vi "Configure Stream U3.vi"(4 "Scan List (-)":u8[](array[numeric])=[31, 31, 31, 31, 31, 31, 31, 31, 31, 31, 31, 31, 31, 31, 31, 31, 31, 31, 31, 31, 31, 31, 31, 31, 31, 31, 31, 31, 31, 31, 31, 31, 31, 31, 31, 31, 31, 31, 31, 31, 31, 31, 31, 31, 31, 31, 31, 31, 31, 31, 31, 31, 31, 31, 31, 31, 31, 31, 31, 31, 31, 31, 31, 31, 31, 31, 31, 31, 31, 31, 31, 31, 31, 31, 31, 31, 31, 31, 31, 31, 31, 31, 31, 31, 31, 31, 31, 31, 31, 31, 31, 31, 31, 31, 31, 31, 31, 31, 31, 31, 31, 31, 31, 31, 31, 31, 31, 31, 31, 31, 31, 31, 31, 31, 31, 31, 31, 31, 31, 31, 31, 31, 31, 31, 31, 31, 31, 31], 6 "Wait Mode":string="LJ_swNONE", 7 "PC buffer size (seconds)":dbl=5.0 format="%.2f", 8 "error in":errorcluster, 9 "Scan List (+)":u8[](array[numeric])=[0, 1, 2, 3], 10 "Scan Rate (Hz)":dbl=1000.0 format="%.2f", 11 "Handle In":i32) -> (0 "error out":errorcluster, 2 "PC buffer size (samples)":i32=5, 3 "Handle Out":i32)   [LabVIEW 2021]
panel:
  # "The + scan list is the positive\nchannels.  For each element in\nthe + list, there must also be\nan element in the - list, which is\nthe negative channels.  For\nsingle-ended channels, put in\n31 for the negative channel."
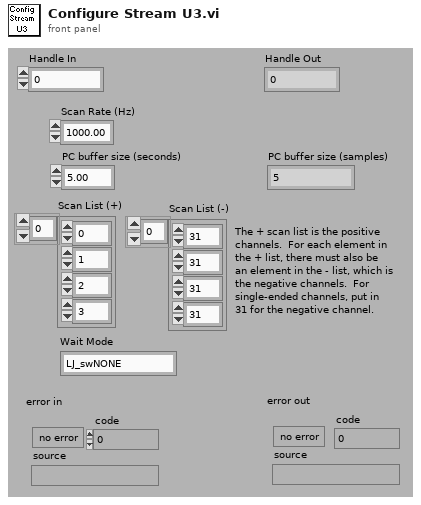
[diagram p1: front panel]
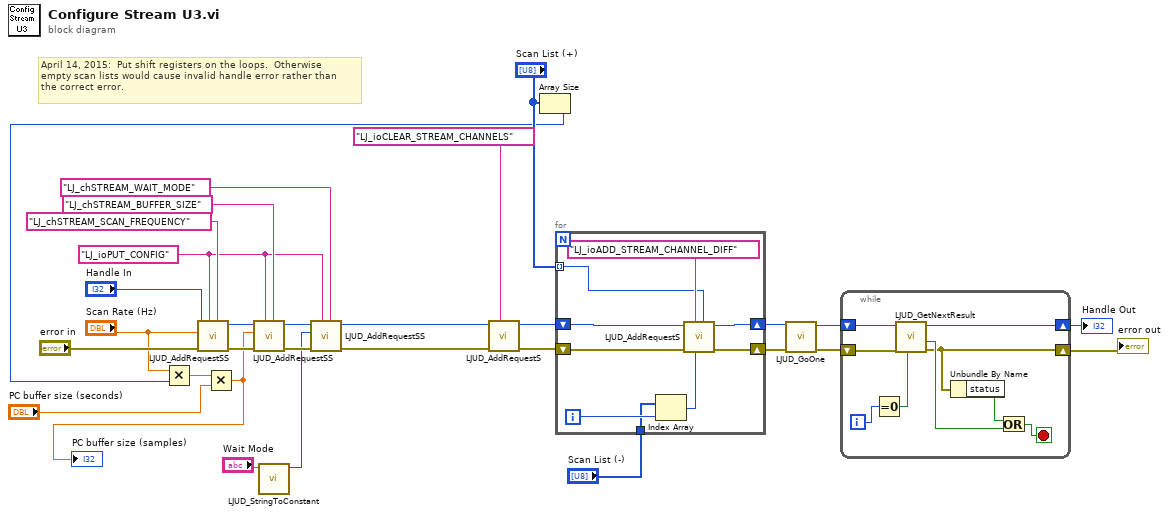
[diagram p0: block diagram]
diagram:
  w9 = "LJ_ioPUT_CONFIG" ("IOType")
  # "April 14, 2015:  Put shift registers on the loops.  Otherwise\nempty scan lists would cause invalid handle error rather than\nthe correct error."
  n1 = call "LJUD_AddRequestSS.vi"("Channel"="LJ_chSTREAM_SCAN_FREQUENCY" ("IOType"), "IOType"=w9, "error in"="error in", "Value"="Scan Rate (Hz)", "Handle In"="Handle In") -> ("error out"=w26:errorcluster, "Handle Out"=w28:i32)  [unwired: 5 in]
  n2 = call "LJUD_StringToConstant.vi"("String"="Wait Mode") -> ("Constant Number"=w7:i32)  [unwired: 9 in, 1 out]
  n3 = Array Size(array="Scan List (+)") -> (size(s)=w11:i32)
  n4 = Multiply(x="Scan Rate (Hz)", y=w11) -> (x*y=w16:dbl)
  n5 = Multiply(x=w16, y="PC buffer size (seconds)") -> (x*y=w4:dbl)
  "PC buffer size (samples)" <- w4
  n6 = call "LJUD_AddRequestSS.vi"("Channel"="LJ_chSTREAM_BUFFER_SIZE" ("IOType"), "IOType"=w9, "error in"=w26, "Value"=w4, "Handle In"=w28) -> ("error out"=w25:errorcluster, "Handle Out"=w27:i32)  [unwired: 5 in]
  n7 = call "LJUD_AddRequestSS.vi"("Channel"="LJ_chSTREAM_WAIT_MODE" ("IOType"), "IOType"=w9, "error in"=w25, "Value"=w7, "Handle In"=w27) -> ("error out"=w2:errorcluster, "Handle Out"=w3:i32)  [unwired: 5 in]
  n8 = call "LJUD_AddRequestS.vi"("IOType"="LJ_ioCLEAR_STREAM_CHANNELS", "error in"=w2, "Handle In"=w3) -> ("error out"=w14:errorcluster, "Handle Out"=w15:i32)  [unwired: 7 in]
  n9 = for {
    shift-right: [w36] -> w20
    shift-left: w14 -> [w37]
    tunnel: "Scan List (+)" -> [w34] mode=indexing
    tunnel: "Scan List (-)" -> [w32]
    shift-right: [w35] -> w21
    shift-left: w15 -> [w39]
    i -> [w33]
    n10 = Index Array(array=w32, index=w33) -> (element=w31:u8)
    n11 = call "LJUD_AddRequestS.vi"("Channel"=w34, "x1"=w31, "IOType"="LJ_ioADD_STREAM_CHANNEL_DIFF", "error in"=w37, "Handle In"=w39) -> ("error out"=w36:errorcluster, "Handle Out"=w35:i32)  [unwired: 5 in]
  }
  n12 = call "LJUD_GoOne.vi"("error in"=w20, "Handle In"=w21) -> ("error out"=w6:errorcluster, "Handle Out"=w18:i32)  [unwired: 8 in]
  n13 = while {
    shift-left: w6 -> [w41]
    shift-right: [w40] -> w5
    shift-right: [w44] -> w19
    shift-left: w18 -> [w46]
    i -> [w43]
    stop <- w48 stop-if-true
    n14 = Equal To 0?(x=w43) -> (x = 0?=w47:bool)
    n15 = call "LJUD_GetNextResult.vi"("GetFirst"=w47, "error in"=w41, "Handle In"=w46) -> ("error out"=w40:errorcluster, "LJE_NO_MORE_DATA_AVAILABLE"=w42:bool, "Handle Out"=w44:i32)  [unwired: 3 in, 3 out]
    n16 = Unbundle By Name(w40) -> ("status"=w45:bool)
    n17 = Or(x=w45, y=w42) -> (x .or. y?=w48:bool)
  }
  "Handle Out" <- w19
  "error out" <- w5
